vi "vi_serial_Bun.vi"() -> ()   [LabVIEW 2021]
uses:
  Program Files (x86)/National Instruments/LabVIEW 2021/examples/Instrument IO/Serial/support/Serial - Settings.ctl
  <vilib>/Instr/_visa.llb/VISA Configure Serial Port (Instr).vi
panel:
  out "output waveform":waveform(i32)(graph)
  out "Waveform Chart":i32[](graph)
  in  "index":i32
  in  "dt":dbl
  out "output array 2":i32[](array[numeric])
  out "Number":i32
  out "message":string=" INSTRUCTIONS:\r\rNormal Use:  When using subVIs that incorporate the error in/error out (or error I/O) structure, place this handler where you want to inform the user of an error, typically at the end of the I/O data path, as the last action of the program.  If the error in error? is ERROR, the handler creates a message describing the error and its source.  If the type of dialog = 1 (default), the message is displayed to the user, who can only acknowedge it.  If the type = 2, the user can acknowledge the message or abort execution; aborting a program with active I/O is not recommended.  If the type = 0, no message is displayed; this is used to process the error programmatically, and the error out cluster elements are wired to individual terminals for that reason.  \r\rOther Use:\n\r\nlocal testing.  To test the error code of a subVI or function that does not have the error I/O structure, you can wire its error code and a source string to the local error code and error source inputs.  If error in error? indicates no error and error code is not equal to 0, the local code and source are substituted for the error in values, and error? is set TRUE (ERROR)."
  in  "Enable Reading":bool
  out "Read Buffer":string
  out "read buffer 2":string
  out "Size of data":u32
  in  "String":string
  out "Result String":string
  in  "stop":bool
  in  "Enable Character Return":bool
  in  "Serial Settings":T1={"baud rate"=115200, "data bits"=8, "parity"=enum."None", "stop bits"=10, "flow control"=0} {"flow control" items=["None"=0, "XON/XOFF"=1, "RTS/CTS"=2, "DTR/DSR"=4]; "stop bits" items=["1.0"=10, "1.5"=15, "2.0"=20]; "data bits" min=5 max=8 step=1; "baud rate" items=["75"=75, "110"=110, "134"=134, "150"=150, "300"=300, "600"=600, "1200"=1200, "1800"=1800, "2400"=2400, "4800"=4800, "7200"=7200, "9600"=9600, "14400"=14400, "19200"=19200, "28800"=28800, "38400"=38400, "56000"=56000, "57600"=57600, "115200"=115200, "128000"=128000, "230400"=230400]}
  in  "VISA resource name":refnum<visa-resource-name>
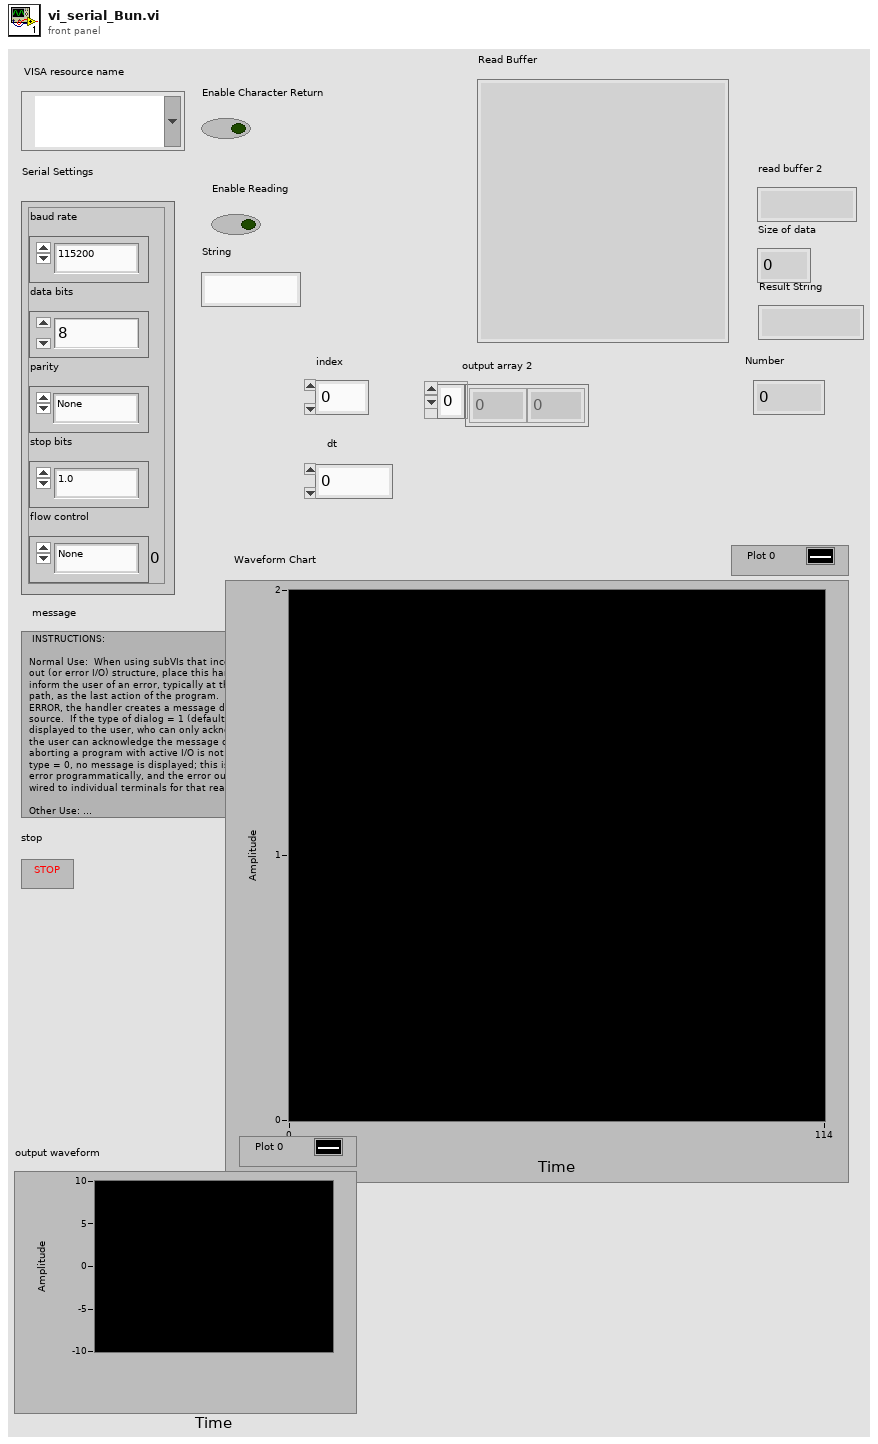
[diagram p1: front panel]
types:
  T1 = typedef "Serial - Settings.ctl" = cluster{"baud rate":u32, "data bits":u16, "parity":enum16{"None", "Odd", "Even", "Mark", "Space"}, "stop bits":u16, "flow control":u16}
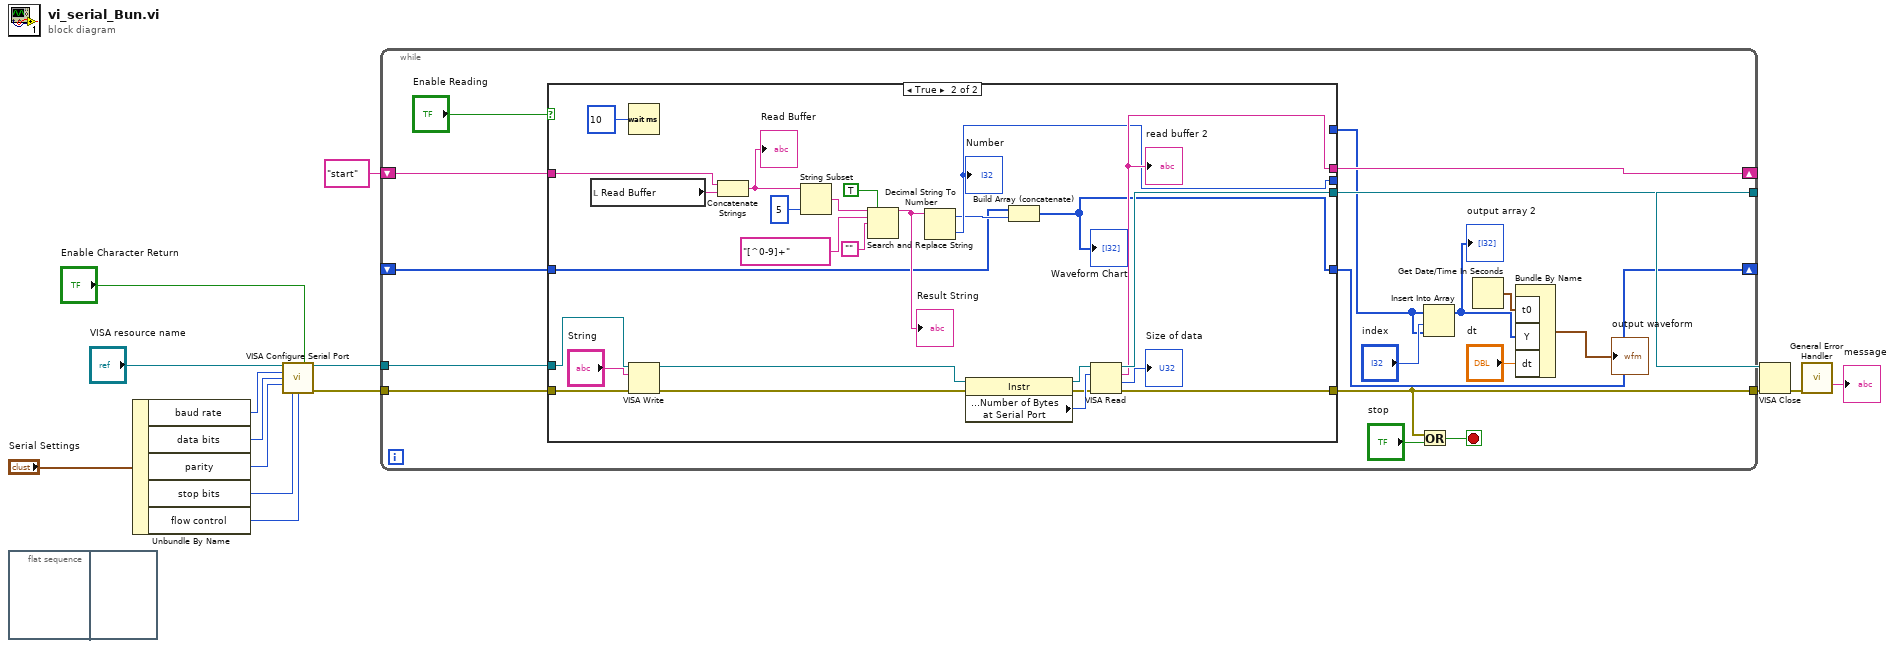
[diagram p0: block diagram]
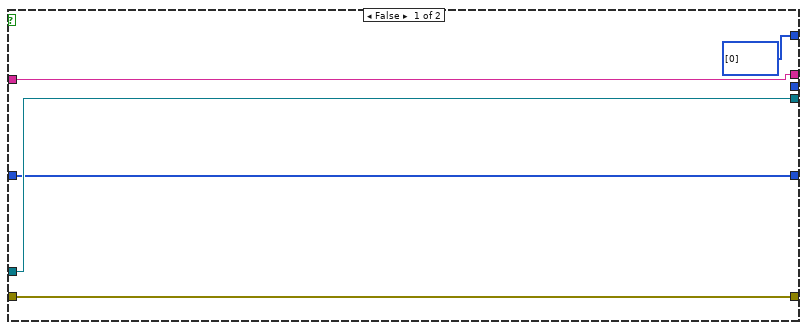
[diagram p2: hidden frame]
diagram:
  n1 = flat-sequence {
    frame #0 {
    }
    frame #1 {
    }
  }
  n2 = Unbundle By Name("Serial Settings") -> ("baud rate"=w14:u32, "data bits"=w13:u16, "parity"=w12:enum16{"None", "Odd", "Even", "Mark", "Space"}, "stop bits"=w11:u16, "flow control"=w10:u16)
  n3 = call-poly "VISA Configure Serial Port"("VISA resource name"="VISA resource name", "Enable Termination\nChar (T)"="Enable Character Return", "baud rate (9600)"=w14, "data bits (8)"=w13, "parity (0:none)"=w12, "stop bits (10: 1 bit)"=w11, "flow control (0:none)"=w10) -> ("VISA resource name out"=w7:refnum<visa-resource-name>, "error out"=w6:errorcluster)  [unwired: 7 in]
  n4 = while {
    tunnel: w7 -> [w32]
    tunnel: w6 -> [w31]
    tunnel: [w23] -> w1
    tunnel: [w30] -> w2
    shift-right: [w25] -> _
    shift-left: "start" ("read buffer") -> [w28]
    shift-right: [w16] -> _
    shift-left: _ -> [w17]
    stop <- w29 stop-if-true
    n5 = case shown="True" "Enable Reading" {
      tunnel: w32 -> [w37 w63]
      tunnel: w31 -> [w36 w62]
      tunnel: [w37 w61] -> w30
      tunnel: [w36 w60] -> w23
      tunnel: [w35 w54] -> w25
      tunnel: w28 -> [w35 w58]
      tunnel: [i32[] [0] _] -> w20
      tunnel: [_ w46] -> _
      tunnel: w17 -> [w33 w38]
      tunnel: [w33 w44] -> w16
      frame False {
      }
      frame True {
        n6 = local read "Read Buffer"() -> (w59:string)
        n7 = Wait (ms)(milliseconds to wait=u32 10) -> ()  [unwired: 1 out]
        n8 = VISA Write(VISA resource name=w63, write buffer="String", error in (no error)=w62) -> (VISA resource name out=w42:refnum<visa-resource-name>, error out=w41:errorcluster)  [unwired: 1 out]
        n9 = Concatenate Strings(w58, w59) -> (w49:string)
        "Read Buffer" <- w49
        n10 = String Subset(string=w49, length (rest)=5 ("length (rest)")) -> (substring=w48:string)  [unwired: 1 in]
        n11 = Search and Replace String(replace all?=TRUE ("replace all? (F)"), input string=w48, search string="[^0-9]+", replace string="") -> (result string=w50:string)  [unwired: 4 in, 3 out]
        "Result String" <- w50
        n12 = Decimal String To Number(string=w50) -> (offset past number=w45:i32, number=w46:i32)  [unwired: 2 in]
        "Number" <- w46
        n13 = property class="Instr"(reference=w42, error in=w41) -> (reference out=w40:refnum<visa-resource-name>, error out=w39:errorcluster, "Serial Settings:Number of Bytes at Serial Port"=w43:u32)
        n14 = Build Array (concatenate)(w38, w45) -> (w44:i32[])
        "Waveform Chart" <- w44
        n15 = VISA Read(VISA resource name=w40, byte count=w43, error in (no error)=w39) -> (VISA resource name out=w61:refnum<visa-resource-name>, read buffer=w54:string, return count=→"Size of data":u32, error out=w60:errorcluster)
        "read buffer 2" <- w54
      }
    }
    n16 = Or(x=w23, y="stop") -> (x .or. y?=w29:bool)
    n17 = Insert Into Array(array=w20, index="index", new element=w20) -> (w22:i32[])
    "output array 2" <- w22
    n18 = Get Date/Time In Seconds() -> (seconds since 1Jan1904=w19:timestamp)
    n19 = Bundle By Name("t0"=w19, "Y"=w22, "dt"="dt") -> (→"output waveform":waveform(i32))  [unwired: 1 in]
  }
  n20 = VISA Close(VISA resource name=w2, error in (no error)=w1) -> (error out=w4:errorcluster)
  n21 = call <vilib>:"General Error Handler.vi"("error in (no error)"=w4) -> ("message"=→"message":string)  [unwired: 10 in, 4 out]
